vi "SetUpSystemDefinitionReferences.vi"(6 "path root vi ref (calling vi)":refnum<vi>, 8 "error in":errorcluster, 10 "Relative Path to SysDef":path, 11 "VeriStandScriptingTestCase in":refnum<class "VeriStandScriptingTestCase.lvclass">) -> (0 "error out":errorcluster, 3 "VeriStandScriptingTestCase out":refnum<class "VeriStandScriptingTestCase.lvclass">)   [LabVIEW 2017, in "VeriStandScriptingTestCase.lvclass"]
uses:
  VeriStandScriptingTestCase.lvclass
  VeriStandScriptingTestCase.lvclass/VeriStandScriptingTestCase.ctl
  <userlib>/_OpenG.lib/file/file.llb/Append Path to Root if Relative - Scalar__ogtk.vi
  VeriStandTestUtilities/VeriStandTestUtilities.lvlib
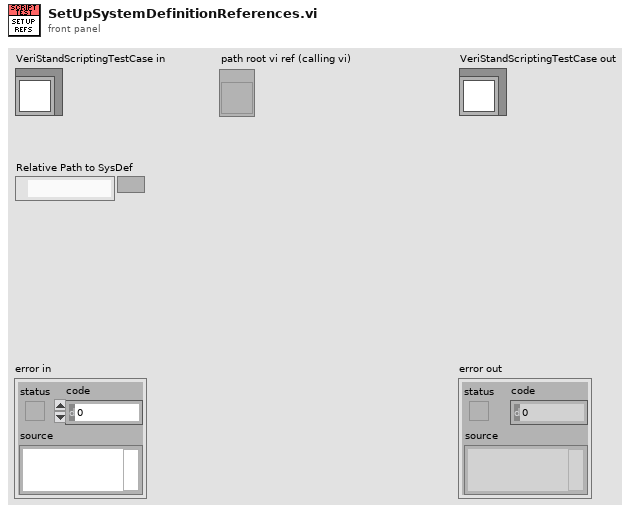
[diagram p1: front panel]
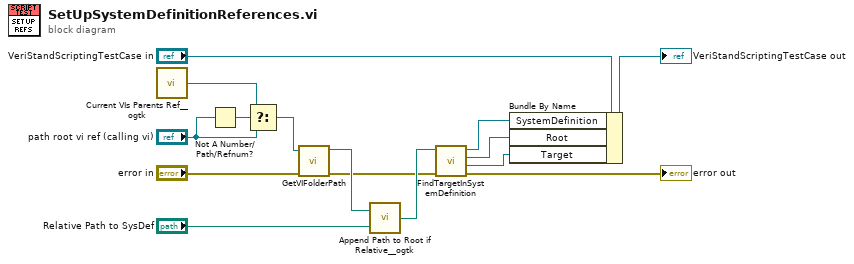
[diagram p0: block diagram]
diagram:
  n1 = call <userlib>:"Current VIs Parents Ref__ogtk.vi"() -> ("Calling VI's Reference"=w5:refnum<vi>)  [unwired: 2 in]
  n2 = Not A Number/Path/Refnum?(number/path/refnum="path root vi ref (calling vi)") -> (NaN/Path/Refnum?=w2:bool)
  n3 = Select(t=w5, s=w2, f="path root vi ref (calling vi)") -> (s? t:f=w1:refnum<vi>)
  n4 = call "GetVIFolderPath.vi"("error in (no error)"="error in", "VI Reference in"=w1) -> ("error out"=w3:errorcluster, "VI Folder Path out"=w15:path)  [unwired: 8 in]
  n5 = call-poly <userlib>:"Append Path to Root if Relative__ogtk.vi"("Absolute or Relative Path"="Relative Path to SysDef", "Root Path"=w15) -> ("Absolute or Appended Path"=w13:path)
  n6 = call "FindTargetInSystemDefinition.vi"("error in"=w3, "system definition path"=w13) -> ("error out"=→"error out":errorcluster, "Target"=w10:refnum<k24>, "Root"=w11:refnum<k24>, "System Definition"=w12:refnum<k24>)  [unwired: 6 in]
  n7 = Bundle By Name(cluster="VeriStandScriptingTestCase in", "SystemDefinition"=w12, "Root"=w11, "Target"=w10) -> (→"VeriStandScriptingTestCase out":refnum<class "VeriStandScriptingTestCase.lvclass">)
